vi "1553B_RECV_fifo.vi"(8 "错误输入（无错误）":errorcluster, 11 "VISA资源名称输入":refnum<visa-resource-name>) -> (0 "error out 2":errorcluster, 3 "VISA资源名称输出":refnum<visa-resource-name>)   [LabVIEW 2012]
uses:
  <vilib>/GPower/VIRegister/Library/Convert/ToU32.vi
  <vilib>/GPower/VIRegister/Library/Convert/ToU8.vi
  <vilib>/GPower/VIRegister/Library/SubVIs/FindRegisterData.vi
  <vilib>/GPower/VIRegister/Library/SubVIs/ReadSub.vi
  <vilib>/GPower/VIRegister/Library/SubVIs/WriteSub.vi
  <vilib>/GPower/VIRegister/Library/QManager/GetRegisterData.vi
  <vilib>/GPower/Error/Library/SetError.vi
  <vilib>/GPower/Error/Library/FilterCodes.vi
  <vilib>/GPower/Error/Library/Filter/FilterMulti.vi
  <vilib>/GPower/VIRegister/Library/QManager/QManagerAction.vi
  <vilib>/GPower/Error/Library/ErrorType.vi
  <vilib>/GPower/Error/Library/SplitAppended.vi
  <vilib>/GPower/Error/Library/SubVIs/ExplanationToError.vi
  <vilib>/GPower/VIRegister/Library/QManager/GetQName.vi
  <vilib>/GPower/VIRegister/Library/QManager/StartQManager.vi
  <vilib>/Utility/error.llb/Trim Whitespace.vi
  <vilib>/dlg_ctls.llb/Space Constant.vi
  <vilib>/Utility/error.llb/Error Code Database.vi
  <vilib>/GPower/Error/Library/SubVIs/SetStatus.vi
  <vilib>/GPower/Error/Library/AppendErrors.vi
  <vilib>/GPower/Error/Library/Append/AppendSingle.vi
  <vilib>/GPower/VIRegister/VIRegister.lvlib
panel:
  out "U8":u8[](array[numeric]) format="%.0x"
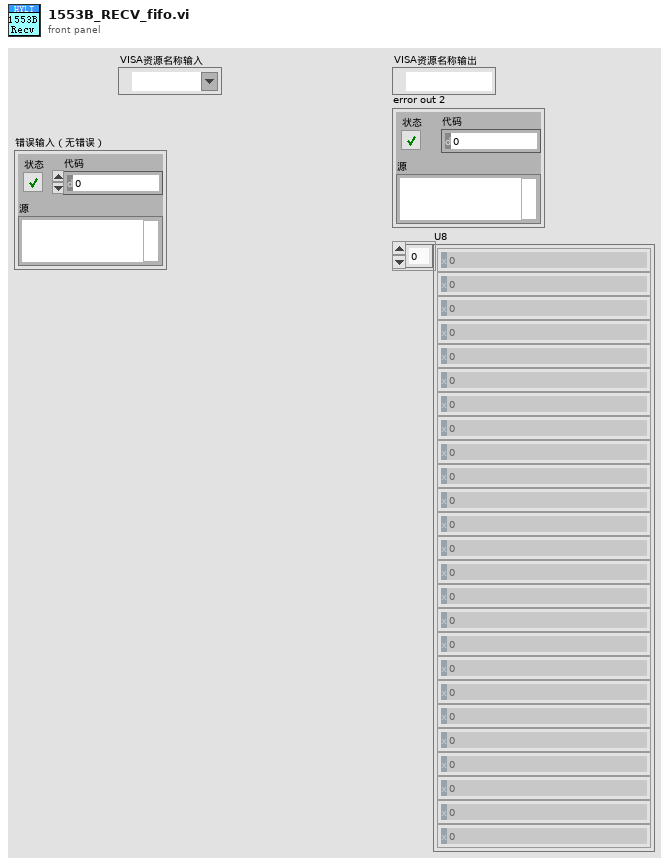
[diagram p1: front panel]
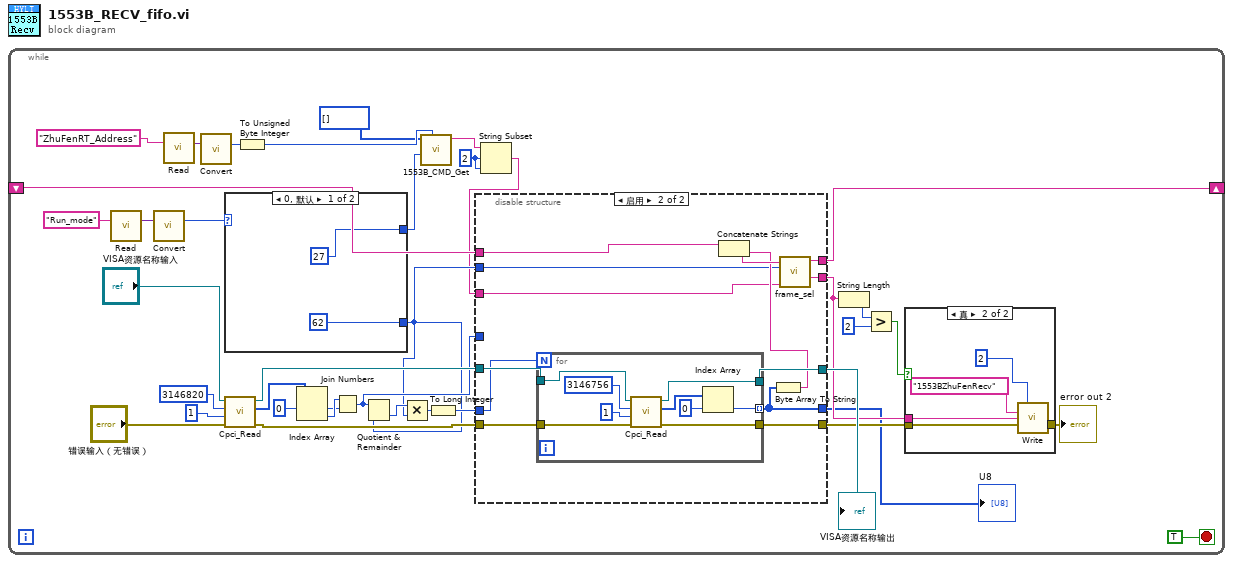
[diagram p0: block diagram]
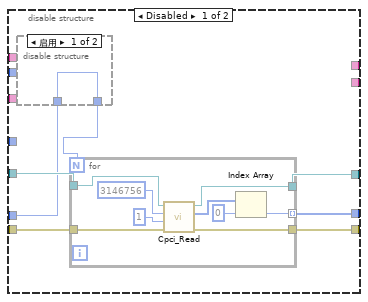
[diagram p3: hidden frame]
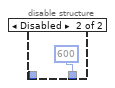
[diagram p4: hidden frame]
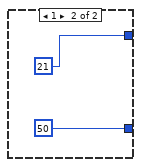
[diagram p5: hidden frame]
diagram:
  n1 = while {
    shift-right: [w17] -> _
    shift-left: _ -> [w16]
    stop <- TRUE stop-if-true
    w10 = 2 ("偏移量(0)")
    n2 = call <vilib>:"Read.vi"("Register name"="Run_mode") -> ("Register value"=w23:variant)  [unwired: 11 in, 3 out]
    n3 = call-poly <vilib>:"Convert.vi"("Register value in"=w23) -> ("Register value out"=w22:u8)  [unwired: 13 in, 1 out]
    n4 = call <vilib>:"Read.vi"("Register name"="ZhuFenRT_Address") -> ("Register value"=w6:variant)  [unwired: 11 in, 3 out]
    n5 = call-poly <vilib>:"Convert.vi"("Register value in"=w6) -> ("Register value out"=w7:u32)  [unwired: 13 in, 1 out]
    n6 = case shown="0, 默认" w22 {
      tunnel: [u16 62 ("y") u16 50 ("y")] -> w11
      tunnel: [u16 27 ("y") u16 21 ("y")] -> w2
      frame 0, Default {
      }
      frame 1 {
      }
    }
    n7 = call "Cpci_Read.vi"("错误输入（无错误）"="错误输入（无错误）", "u32_len"=1, "基地址"=u32 3146820, "VISA资源名称"="VISA资源名称输入") -> ("错误输出"=w25:errorcluster, "U8"=w33:u8[], "VISA资源名称输出"=w27:refnum<visa-resource-name>)  [unwired: 5 in]
    n8 = To Unsigned Byte Integer(number=w7) -> (unsigned 8bit integer=w8:u8)
    n9 = Index Array(array=w33, index #1=0 ("索引")) -> (element #1=w30:u8, element #2=w31:u8)  [unwired: 1 in]
    n10 = Join Numbers(hi=w31, lo=w30) -> ((hi.lo)=w18:u16)
    n11 = Quotient & Remainder(x=w18, y=w11) -> (floor(x/y)=w29:u16)  [unwired: 1 out]
    n12 = Multiply(x=w29, y=w11) -> (x*y=w28:u16)
    n13 = call "1553B_CMD_Get.vi"("RT地址(默认：01111)"=w8, "字长"=w2, "数据字数组"=u16[] []) -> ("1553B指令"=w9:string)  [unwired: 8 in]
    n14 = To Long Integer(number=w28) -> (32bit integer=w20:i32)
    n15 = String Subset(string=w9, offset (0)=w10, length (rest)=w10) -> (substring=w3:string)
    n16 = disable-structure shown="启用" {
      disable-tunnel: w27 -> [w51 w75]
      disable-tunnel: [w50 w71] -> w1
      disable-tunnel: [w49 w74] -> w26
      disable-tunnel: w25 -> [w48 w73]
      disable-tunnel: [w47 w72] -> w24
      disable-tunnel: w20 -> [w46 w63]
      disable-tunnel: w18 -> [_ _]
      disable-tunnel: [_ w67] -> w15
      disable-tunnel: [_ w66] -> w17
      disable-tunnel: w16 -> [_ w69]
      disable-tunnel: w11 -> [_ w65]
      disable-tunnel: w3 -> [_ w64]
      frame Disabled {
        n17 = disable-structure shown="启用" {
          disable-tunnel: w46 -> [w52 _]
          disable-tunnel: [w52 600] -> w45
          frame Enabled {
          }
          frame Disabled {
          }
        }
        n18 = for {
          N: w45 -> [_]
          tunnel: w51 -> [w60]
          tunnel: [w54] -> w50 mode=indexing
          tunnel: [w59] -> w49
          tunnel: w48 -> [w58]
          tunnel: [w57] -> w47
          n19 = call "Cpci_Read.vi"("错误输入（无错误）"=w58, "u32_len"=1, "基地址"=u32 3146756, "VISA资源名称"=w60) -> ("错误输出"=w57:errorcluster, "U8"=w56:u8[], "VISA资源名称输出"=w59:refnum<visa-resource-name>)  [unwired: 5 in]
          n20 = Index Array(array=w56, index=0 ("索引")) -> (element=w54:u8)
        }
      }
      frame Enabled {
        n21 = for {
          N: w63 -> [_]
          tunnel: w75 -> [w82]
          tunnel: [w76] -> w71 mode=indexing
          tunnel: [w81] -> w74
          tunnel: w73 -> [w80]
          tunnel: [w79] -> w72
          n22 = call "Cpci_Read.vi"("错误输入（无错误）"=w80, "u32_len"=1, "基地址"=u32 3146756, "VISA资源名称"=w82) -> ("错误输出"=w79:errorcluster, "U8"=w78:u8[], "VISA资源名称输出"=w81:refnum<visa-resource-name>)  [unwired: 5 in]
          n23 = Index Array(array=w78, index=0 ("索引")) -> (element=w76:u8)
        }
        n24 = Byte Array To String(unsigned byte array=w71) -> (string=w68:string)
        n25 = Concatenate Strings(w69, w68) -> (w70:string)
        n26 = call "frame_sel.vi"("正则表达式"=w64, "帧长"=w65, "输入字符串"=w70) -> ("结果"=w67:string, "剩余"=w66:string)  [unwired: 7 in]
      }
    }
    "VISA资源名称输出" <- w26
    "U8" <- w1
    n27 = String Length(string=w15) -> (length=w14:i32)
    n28 = Greater?(x=w14, y=2) -> (0:w12:bool)
    n29 = case shown="真" w12 {
      tunnel: [w39 w44] -> w37
      tunnel: w24 -> [w39 w41]
      tunnel: w15 -> [_ w40]
      frame False {
      }
      frame True {
        n30 = call <vilib>:"Write.vi"("Timeout"=2, "Register name"="1553BZhuFenRecv", "Register value"=w40, "Error in"=w41) -> ("Error out"=w44:errorcluster)  [unwired: 9 in, 2 out]
      }
    }
    "error out 2" <- w37
  }
